vi "gds_transmitter.vi"(8 "error in (no error)":errorcluster, 11 "Modulation Parameters":T1) -> (0 "error out":errorcluster, 1 "Symbols Out":cdb[](array[numeric]) caption="symbols out" format="%.2f", 2 "Key Bit Sequence":i8[](array[numeric]), 3 "Transmitted Signal":T2 {"Y" format="%.3f"; "dt" format="%^.2e"; "t0" format="%.4f"})   [LabVIEW 2012]
uses:
  <vilib>/addons/Modulation/Analog/controls/Complex Data Waveform.ctl
  <vilib>/addons/Modulation/niAMT.lvlib
panel:
  out "Preamble":i8[](array[numeric])
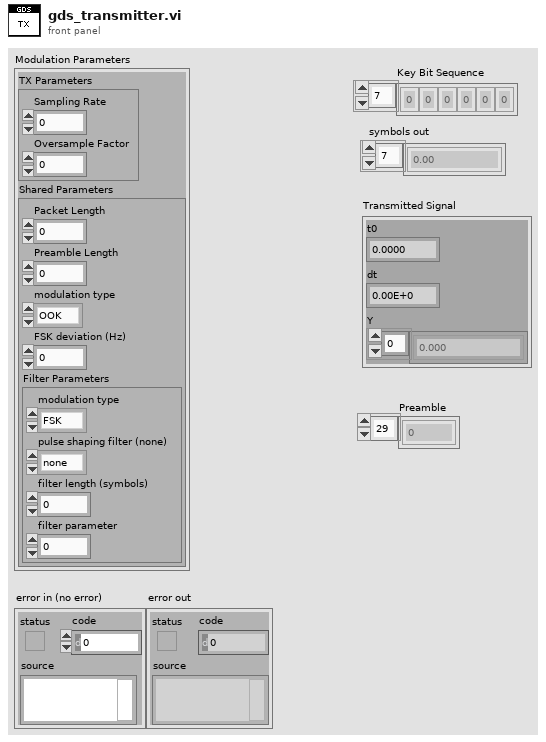
[diagram p1: front panel]
types:
  T1 = cluster{"TX Parameters":cluster{"Sampling Rate":dbl, "Oversample Factor":i32}, "Shared Parameters":cluster{"Packet Length":i32, "Preamble Length":i32, "modulation type":enum16{"OOK", "FSK", "PSK", "QAM", "MSK", "PAM", "ASK", "CPM"}, "FSK deviation (Hz)":dbl, "Filter Parameters":cluster{"modulation type":enum16{"FSK", "PSK", "QAM", "MSK", "PAM", "ASK", "CPM"}, "pulse shaping filter (none)":enum16{"none", "Raised Cosine", "Root Raised Cos", "Gaussian"}, "filter length (symbols)":i32, "filter parameter":dbl}}}
  T2 = typedef "niAMT.lvlib/Complex Data Waveform.ctl" = cluster{"t0":dbl, "dt":dbl, "Y":cdb[]}
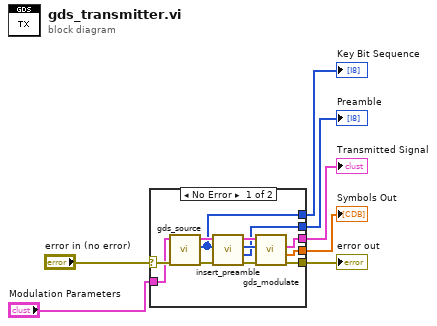
[diagram p0: block diagram]
diagram:
  n1 = case shown="No Error" "error in (no error)" {
    selector: "error in (no error)" -> [w19 w20]
    tunnel: [w18 w20] -> w6
    tunnel: [w12 _] -> w5
    tunnel: [w11 _] -> w4
    tunnel: "Modulation Parameters" -> [w15 _]
    tunnel: [w10 _] -> w2
    tunnel: [w8 _] -> w1
    frame No Error {
      n2 = call "gds_source.vi"("error in (no error)"=w19, "Modulation Parameters In"=w15) -> ("error out"=w17:errorcluster, "Key Bit Sequence"=w10:i8[], "Modulation Parameters Out"=w14:T1)  [unwired: 7 in]
      n3 = call "insert_preamble.vi"("error in (no error)"=w17, "Payload"=w10, "Modulation Parameters In"=w14) -> ("error out"=w16:errorcluster, "Preamble"=w8:i8[], "Transmitted Bit Sequence"=w9:i8[], "Modulation Parameters  Out"=w13:T1)  [unwired: 5 in]
      n4 = call "gds_modulate.vi"("error in (no error)"=w16, "input bit stream"=w9, "Modulation Parameters"=w13) -> ("error out"=w18:errorcluster, "symbols out"=w11:cdb[], "output complex waveform"=w12:T2)  [unwired: 5 in, 1 out]
    }
    frame Error {
    }
  }
  "Key Bit Sequence" <- w2
  "error out" <- w6
  "Transmitted Signal" <- w5
  "Symbols Out" <- w4
  "Preamble" <- w1
